vi "PID Get Error (DBL Array).vi"(0 "setpoint":dbl[](array[numeric])=[0.0] format="%.2f", 1 "process variable":dbl[](array[numeric])=[0.0] format="%.2f", 2 "beta":dbl[](array[numeric])=[1.0] format="%.2f", 3 "linearity":dbl[](array[numeric])=[1.0] format="%.2f", 4 "setpoint range":T1(array[cluster])=[{"setpoint high"=100.0, "setpoint low"=0.0}] {"setpoint high" format="%.2f"; "setpoint low" format="%.2f"}) -> (5 "error (with beta)":dbl[](array[numeric]) format="%.2f", 6 "error":dbl[](array[numeric]) format="%.2f")   [LabVIEW 2020, in "NI_PID_pid.lvlib"]
doc: "This function calculates the error between the process variable and setpoint value. The error (with beta) output is used for the proportional action and the error output is used for the integral action."
uses:
  NI_PID_pid.lvlib
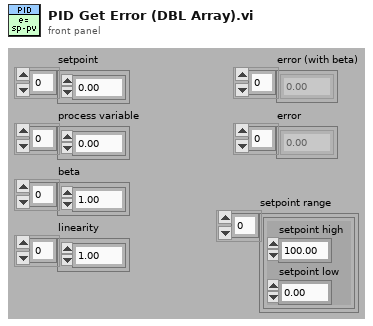
[diagram p1: front panel]
types:
  T1 = cluster{"setpoint high":dbl, "setpoint low":dbl}[]
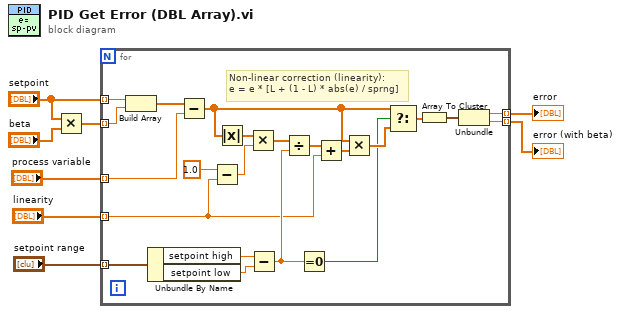
[diagram p0: block diagram]
diagram:
  n1 = Multiply(x="setpoint", y="beta") -> (x*y=w8:dbl[])
  n2 = for {
    tunnel: w8 -> [w29] mode=indexing
    tunnel: "setpoint" -> [w14] mode=indexing
    tunnel: "process variable" -> [w13] mode=indexing
    tunnel: "linearity" -> [w12] mode=indexing
    tunnel: "setpoint range" -> [w11] mode=indexing
    tunnel: [w10] -> w2 mode=indexing
    tunnel: [w9] -> w1 mode=indexing
    # "Non-linear correction (linearity):\ne = e * [L + (1 - L) * abs(e) / sprng]"
    n3 = Build Array(w14, w29) -> (w28:dbl[])
    n4 = Unbundle By Name(w11) -> ("setpoint high"=w16:dbl, "setpoint low"=w15:dbl)
    n5 = Subtract(x=w28, y=w13) -> (x-y=w19:dbl[])
    n6 = Subtract(x=1.0, y=w12) -> (x-y=w26:dbl)
    n7 = Absolute Value(x=w19) -> (abs(x)=w27:dbl[])
    n8 = Multiply(x=w27, y=w26) -> (x*y=w25:dbl[])
    n9 = Subtract(x=w16, y=w15) -> (x-y=w21:dbl)
    n10 = Divide(x=w25, y=w21) -> (x/y=w24:dbl[])
    n11 = Equal To 0?(x=w21) -> (x = 0?=w17:bool)
    n12 = Add(x=w24, y=w12) -> (x+y=w23:dbl[])
    n13 = Multiply(x=w19, y=w23) -> (x*y=w18:dbl[])
    n14 = Select(t=w19, s=w17, f=w18) -> (s? t:f=w20:dbl[])
    n15 = Array To Cluster(array=w20) -> (cluster=w22:cluster{"[0]":dbl, "[1]":dbl})
    n16 = Unbundle(w22) -> ("[0]"=w9:dbl, "[1]"=w10:dbl)
  }
  "error" <- w1
  "error (with beta)" <- w2
